vi "Hot Goal Rotation.vi"(1 "Degrees to rotate":dbl=18.6 format="%#_13g", 2 "Rotate Power":dbl=0.3 format="%#_13g") -> ()   [LabVIEW 2013]
uses:
  Robot Global Data.vi
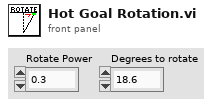
[diagram p1: front panel]
types:
  T1 = typedef "WPI_GyroDevRef.ctl" = cluster{"DevStatus":errorcluster, "Analog Module":T2, "Analog Channel":T3, "Offset":dbl, "Gain (VoltsPerDegree/Second)":dbl}
  T2 = typedef "FPGA_TypedefAnalogModule.ctl" = enum16{"Analog Module 1", "Analog Module 2"}
  T3 = typedef "FPGA_AIChannel.ctl" = enum8{"AI 1", "AI 2", "AI 3", "AI 4", "AI 5", "AI 6", "AI 7", "AI 8", "Invalid"}
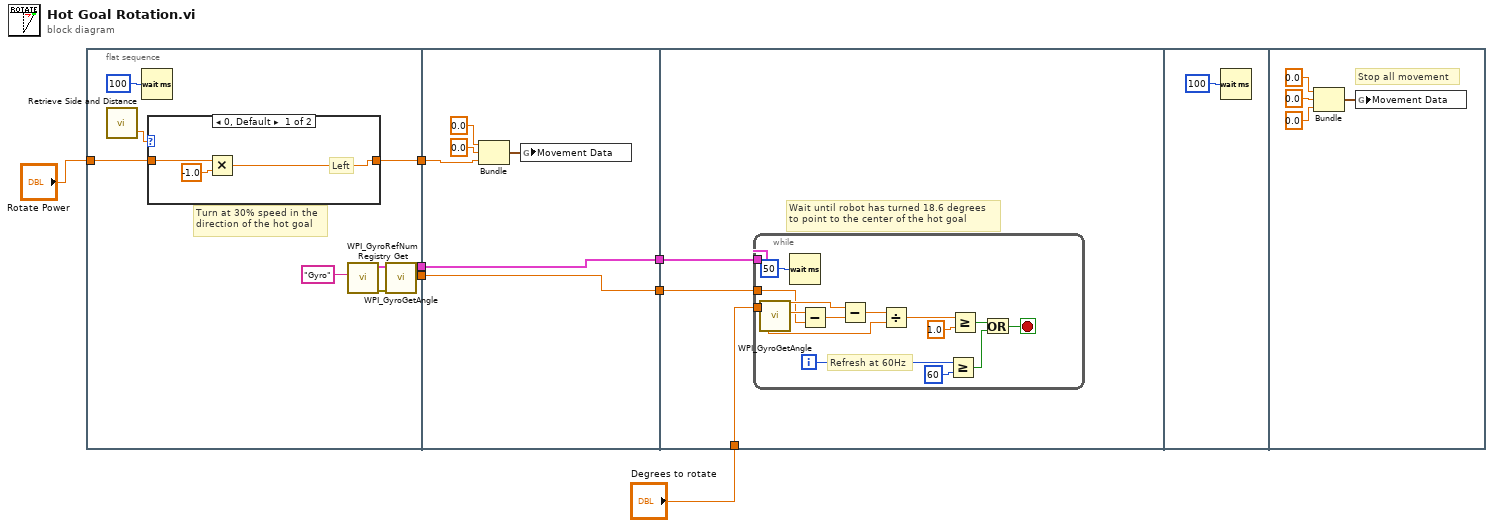
[diagram p0: block diagram]
diagram:
  n1 = flat-sequence {
    tunnel: [w16] -> w7
    tunnel: "Rotate Power" -> [w14]
    tunnel: [w9] -> w3
    tunnel: [w8] -> w2
    tunnel: w7 -> [w23]
    tunnel: [w22] -> w4
    tunnel: w3 -> [w22]
    tunnel: w2 -> [w21]
    tunnel: [w21] -> w1
    tunnel: "Degrees to rotate" -> [w29]
    tunnel: w4 -> [w28]
    tunnel: w1 -> [w27]
    frame #0 {
      # "Turn at 30% speed in the\ndirection of the hot goal"
      n2 = call "Retrieve Side and Distance.vi"() -> ("Side"=w13:dbl)  [unwired: 2 in, 1 out]
      n3 = Wait (ms)(milliseconds to wait=u32 100) -> ()  [unwired: 1 out]
      n4 = case shown="0, Default" w13 {
        tunnel: [w19 w20] -> w16
        tunnel: w14 -> [w17 w20]
        frame 0, Default {
          # "Left"
          n5 = Multiply(x=w17, y=-1.0) -> (x*y=w19:dbl)
        }
        frame 1 {
          # "Right"
        }
      }
      n6 = call <vilib>:"WPI_GyroRefNum Registry Get.vi"("refnum name"="Gyro") -> ("error out"=w11:errorcluster, "GyroDevRef"=w10:T1)  [unwired: 9 in]
      n7 = call <vilib>:"WPI_GyroGetAngle.vi"("error in (no error)"=w11, "GyroDevRef"=w10) -> ("Angle"=w8:dbl, "GyroDevRef"=w9:T1)  [unwired: 6 in, 2 out]
    }
    frame #1 {
      n8 = Bundle(0.0, 0.0, "Rotate Power"=w23) -> (w26:cluster{dbl, dbl, "Rotate Power":dbl})  [unwired: 1 in]
      n9 = global write "Robot Global Data.vi" "Movement Data"(w26) -> ()
    }
    frame #2 {
      # "Wait until robot has turned 18.6 degrees\nto point to the center of the hot goal"
      n10 = while {
        tunnel: w29 -> [w33]
        tunnel: w28 -> [w37]
        tunnel: w27 -> [w31]
        i -> [w39]
        stop <- w30 stop-if-true
        # "Refresh at 60Hz"
        n11 = call <vilib>:"WPI_GyroGetAngle.vi"("GyroDevRef"=w37) -> ("Angle"=w43:dbl)  [unwired: 7 in, 3 out]
        n12 = Wait (ms)(milliseconds to wait=u32 50) -> ()  [unwired: 1 out]
        n13 = Subtract(x=w43, y=w31) -> (x-y=w32:dbl)
        n14 = Subtract(x=w33, y=w32) -> (x-y=w34:dbl)
        n15 = Divide(x=w34, y=w33) -> (x/y=w35:dbl)
        n16 = Greater Or Equal?(x=w39, y=60) -> (x >= y?=w42:bool)
        n17 = Greater Or Equal?(x=w35, y=1.0) -> (x >= y?=w41:bool)
        n18 = Or(x=w41, y=w42) -> (x .or. y?=w30:bool)
      }
    }
    frame #3 {
      n19 = Wait (ms)(milliseconds to wait=u32 100) -> ()  [unwired: 1 out]
    }
    frame #4 {
      # "Stop all movement"
      n20 = Bundle(0.0, 0.0, 0.0) -> (w48:cluster{dbl, dbl, dbl})  [unwired: 1 in]
      n21 = global write "Robot Global Data.vi" "Movement Data"(w48) -> ()
    }
  }
